vi "ConfigureAdaptorr07.vi"() -> ()   [LabVIEW 2011]
panel:
  in  "Set Point C (Torr)":dbl=20.0
  in  "Trip Point 2 (Torr)":dbl=200.0
  in  "Trip Point 1(Torr)":dbl=700.0
  in  "error":errorcluster
  in  "Set Point D (Torr)":dbl=40.0
  in  "Set Point B (Torr)":dbl=76.0
  in  "Set Point A (Torr)":dbl=10.0
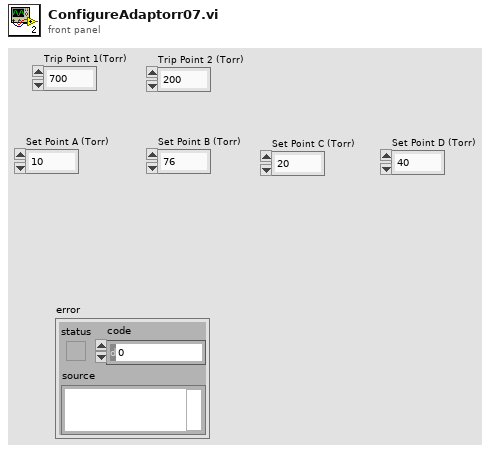
[diagram p1: front panel]
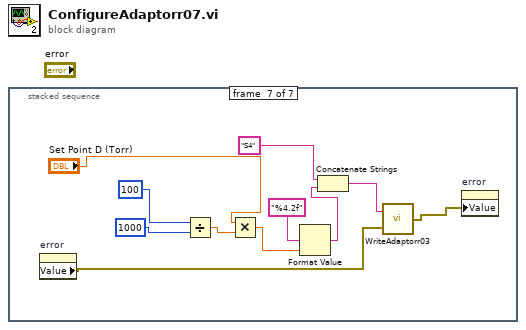
[diagram p0: block diagram]
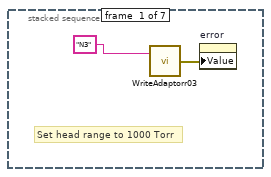
[diagram p2: hidden frame]
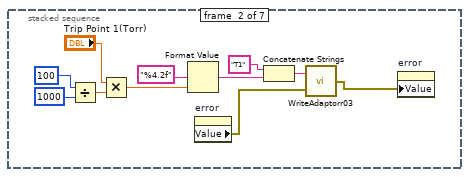
[diagram p3: hidden frame]
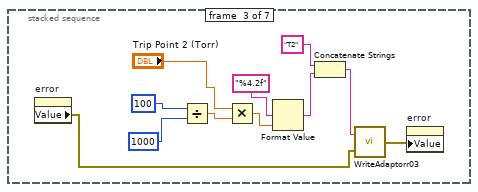
[diagram p4: hidden frame]
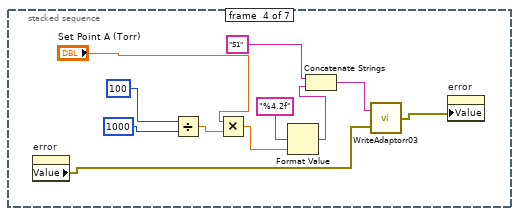
[diagram p5: hidden frame]
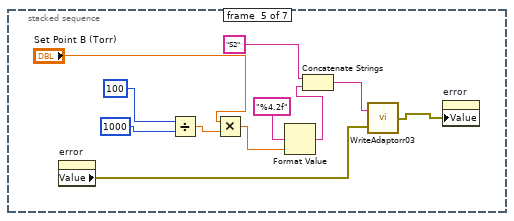
[diagram p6: hidden frame]
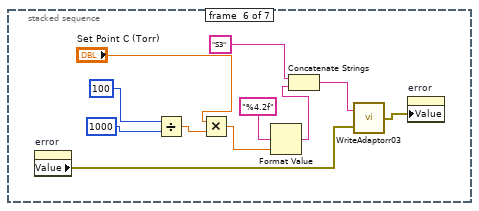
[diagram p7: hidden frame]
diagram:
  n1 = stacked-sequence {
    frame #0 {
      # "Set head range to 1000 Torr"
      n2 = call "WriteAdaptorr03.vi"("string to write"="N3") -> ("error out"=w1:errorcluster)  [unwired: 1 in]
      n3 = property on="error" class="Clust (strict)"("Value"=w1) -> ()  [unwired: 2 in, 2 out]
    }
    frame #1 {
      n4 = Divide(x=100, y=1000) -> (x/y=w11:dbl)
      n5 = Multiply(x="Trip Point 1(Torr)", y=w11) -> (x*y=w6:dbl)
      n6 = Format Value(format string="%4.2f", value (0)=w6) -> (output string=w8:string)  [unwired: 1 in]
      n7 = property on="error" class="Clust (strict)"() -> ("Value"=w4:errorcluster)  [unwired: 2 in, 2 out]
      n8 = Concatenate Strings("T1", w8) -> (w7:string)
      n9 = call "WriteAdaptorr03.vi"("error in (no error)"=w4, "string to write"=w7) -> ("error out"=w3:errorcluster)
      n10 = property on="error" class="Clust (strict)"("Value"=w3) -> ()  [unwired: 2 in, 2 out]
    }
    frame #2 {
      n11 = property on="error" class="Clust (strict)"() -> ("Value"=w15:errorcluster)  [unwired: 2 in, 2 out]
      n12 = Divide(x=100, y=1000) -> (x/y=w22:dbl)
      n13 = Multiply(x="Trip Point 2 (Torr)", y=w22) -> (x*y=w18:dbl)
      n14 = Format Value(format string="%4.2f", value (0)=w18) -> (output string=w16:string)  [unwired: 1 in]
      n15 = Concatenate Strings("T2", w16) -> (w19:string)
      n16 = call "WriteAdaptorr03.vi"("error in (no error)"=w15, "string to write"=w19) -> ("error out"=w14:errorcluster)
      n17 = property on="error" class="Clust (strict)"("Value"=w14) -> ()  [unwired: 2 in, 2 out]
    }
    frame #3 {
      n18 = property on="error" class="Clust (strict)"() -> ("Value"=w26:errorcluster)  [unwired: 2 in, 2 out]
      n19 = Divide(x=100, y=1000) -> (x/y=w30:dbl)
      n20 = Multiply(x="Set Point A (Torr)", y=w30) -> (x*y=w34:dbl)
      n21 = Format Value(format string="%4.2f", value (0)=w34) -> (output string=w35:string)  [unwired: 1 in]
      n22 = Concatenate Strings("S1", w35) -> (w32:string)
      n23 = call "WriteAdaptorr03.vi"("error in (no error)"=w26, "string to write"=w32) -> ("error out"=w25:errorcluster)
      n24 = property on="error" class="Clust (strict)"("Value"=w25) -> ()  [unwired: 2 in, 2 out]
    }
    frame #4 {
      n25 = property on="error" class="Clust (strict)"() -> ("Value"=w37:errorcluster)  [unwired: 2 in, 2 out]
      n26 = Divide(x=100, y=1000) -> (x/y=w44:dbl)
      n27 = Multiply(x="Set Point B (Torr)", y=w44) -> (x*y=w40:dbl)
      n28 = Format Value(format string="%4.2f", value (0)=w40) -> (output string=w39:string)  [unwired: 1 in]
      n29 = Concatenate Strings("S2", w39) -> (w42:string)
      n30 = call "WriteAdaptorr03.vi"("error in (no error)"=w37, "string to write"=w42) -> ("error out"=w36:errorcluster)
      n31 = property on="error" class="Clust (strict)"("Value"=w36) -> ()  [unwired: 2 in, 2 out]
    }
    frame #5 {
      n32 = property on="error" class="Clust (strict)"() -> ("Value"=w48:errorcluster)  [unwired: 2 in, 2 out]
      n33 = Divide(x=100, y=1000) -> (x/y=w55:dbl)
      n34 = Multiply(x="Set Point C (Torr)", y=w55) -> (x*y=w50:dbl)
      n35 = Format Value(format string="%4.2f", value (0)=w50) -> (output string=w49:string)  [unwired: 1 in]
      n36 = Concatenate Strings("S3", w49) -> (w52:string)
      n37 = call "WriteAdaptorr03.vi"("error in (no error)"=w48, "string to write"=w52) -> ("error out"=w47:errorcluster)
      n38 = property on="error" class="Clust (strict)"("Value"=w47) -> ()  [unwired: 2 in, 2 out]
    }
    frame #6 {
      n39 = property on="error" class="Clust (strict)"() -> ("Value"=w60:errorcluster)  [unwired: 2 in, 2 out]
      n40 = Divide(x=100, y=1000) -> (x/y=w66:dbl)
      n41 = Multiply(x="Set Point D (Torr)", y=w66) -> (x*y=w62:dbl)
      n42 = Format Value(format string="%4.2f", value (0)=w62) -> (output string=w61:string)  [unwired: 1 in]
      n43 = Concatenate Strings("S4", w61) -> (w64:string)
      n44 = call "WriteAdaptorr03.vi"("error in (no error)"=w60, "string to write"=w64) -> ("error out"=w59:errorcluster)
      n45 = property on="error" class="Clust (strict)"("Value"=w59) -> ()  [unwired: 2 in, 2 out]
    }
  }
